vi "Check the Digital Unsigned Signed Format of String.vi"(8 "error in (no error)":errorcluster, 10 "Value":string, 11 "DigNum Refnum":refnum<vi>) -> (0 "error out":errorcluster, 2 "Valuse Without Flag":string, 3 "dup DigNum Refnum":refnum<vi>)   [LabVIEW 2021, in "CANOpen Addon System Explorer.lvlib"]
uses:
  CANOpen Addon System Explorer.lvlib
  <vilib>/regexp/Match Regular Expression.xnode
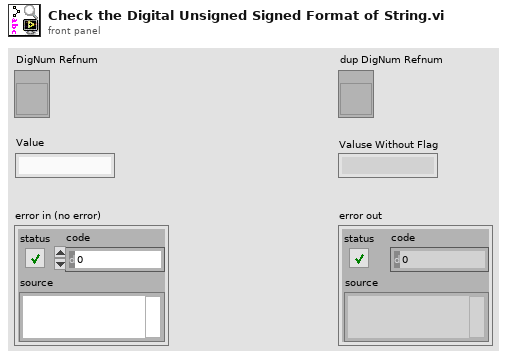
[diagram p1: front panel]
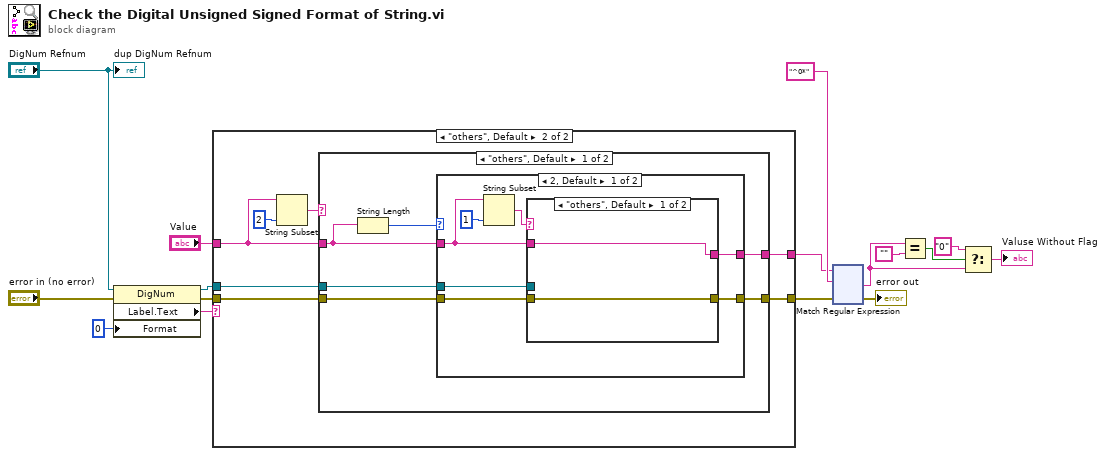
[diagram p0: block diagram]
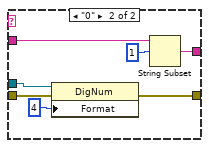
[diagram p3: hidden frame]
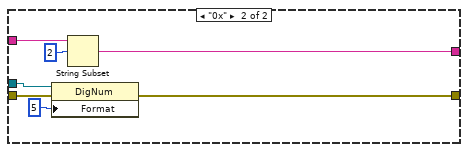
[diagram p5: hidden frame]
diagram:
  n1 = property class="DigNum"(reference="DigNum Refnum", error in="error in (no error)", "Format"=u8 0 ("Display Format:Format")) -> (reference out=w14:refnum<vi>, error out=w13:errorcluster, "Label.Text"=w11:string)
  n2 = case shown="\"others\", Default" w11 {
    tunnel: "Value" -> [w18 w23]
    tunnel: w13 -> [w17 w22]
    tunnel: w14 -> [_ w21]
    tunnel: [w18 w19] -> w7
    tunnel: [w17 w20] -> w9
    frame "CreationDate", "CreationTime", "ModificationDate", "ModificationTime" {
    }
    frame "others", Default {
      n3 = String Subset(string=w23, length (rest)=2 ("length (rest)")) -> (substring=w24:string)  [unwired: 1 in]
      n4 = case shown="\"others\", Default" w24 {
        tunnel: w23 -> [w30 w56]
        tunnel: [w29 w54] -> w19
        tunnel: w22 -> [w28 w53]
        tunnel: [w27 w52] -> w20
        tunnel: w21 -> [w26 w51]
        frame "others", Default {
          n5 = String Length(string=w30) -> (length=w31:i32)
          n6 = case shown="2, Default" w31 {
            tunnel: w30 -> [w36 w49]
            tunnel: [w35 w49] -> w29
            tunnel: w28 -> [w33 w48]
            tunnel: [w32 w48] -> w27
            tunnel: w26 -> [w34 _]
            frame 2, Default {
              n7 = String Subset(string=w36, length (rest)=1 ("length (rest)")) -> (substring=w37:string)  [unwired: 1 in]
              n8 = case shown="\"others\", Default" w37 {
                tunnel: w36 -> [w40 w47]
                tunnel: [w40 w45] -> w35
                tunnel: w34 -> [_ w44]
                tunnel: w33 -> [w39 w43]
                tunnel: [w39 w41] -> w32
                frame "others", Default {
                }
                frame "0" {
                  n9 = property class="DigNum"(reference=w44, error in=w43, "Format"=u8 4 ("Display Format:Format")) -> (error out=w41:errorcluster)  [unwired: 1 out]
                  n10 = String Subset(string=w47, offset (0)=1) -> (substring=w45:string)  [unwired: 1 in]
                }
              }
            }
            frame 1 {
            }
          }
        }
        frame "0x" {
          n11 = property class="DigNum"(reference=w51, error in=w53, "Format"=u8 5 ("Display Format:Format")) -> (error out=w52:errorcluster)  [unwired: 1 out]
          n12 = String Subset(string=w56, offset (0)=2) -> (substring=w54:string)  [unwired: 1 in]
        }
      }
    }
  }
  n13 = xnode "Match Regular Expression"("input string"=w7, "regular expression"="^0*", "error in"=w9) -> ("after match"=w3:string, "error out"=→"error out":errorcluster)  [unwired: 3 in, 3 out]
  n14 = Equal?(x=w3, y="") -> (x = y?=w5:bool)
  n15 = Select(t="0", s=w5, f=w3) -> (s? t:f=→"Valuse Without Flag":string)
  "dup DigNum Refnum" <- "DigNum Refnum"
